vi "batas tanki(SubVI).vi"(11 "Numeric in":dbl) -> (3 "Numeric out":dbl)   [LabVIEW 2017]
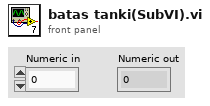
[diagram p1: front panel]
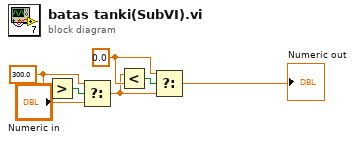
[diagram p0: block diagram]
diagram:
  w6 = 0.0
  w3 = 300.0
  n1 = Greater?(x="Numeric in", y=w3) -> (0:w1:bool)
  n2 = Select(t=w3, s=w1, f="Numeric in") -> (s? t:f=w5:dbl)
  n3 = Less?(x=w5, y=w6) -> (x < y?=w4:bool)
  n4 = Select(t=w6, s=w4, f=w5) -> (s? t:f=→"Numeric out":dbl)
